vi "Measurement Logic.vi"() -> ()   [LabVIEW 2024, in "NIFgenSignalVoltageGeneration.lvlib"]
uses:
  NIFgenSignalVoltageGeneration.lvlib
  Measurement Configuration.ctl
  Measurement Results.ctl
  <vilib>/MeasurementLink/MeasurementLink Measurement Server/Measure Call Context/Measure Call Context.lvclass
  <instrlib>/niFgen/niFgen.llb/niFgen Output Mode.ctl
  <vilib>/MeasurementLink/MeasurementLink niFGEN/Initialize Sessions - 1Sess.vi
  <vilib>/MeasurementLink/MeasurementLink Session Management V1/Session Reservation/Session Reservation.lvclass
  <vilib>/MeasurementLink/MeasurementLink niFGEN/MeasurementLink niFGEN.lvlib
panel:
  out "Generated Waveform":waveform(dbl)(graph)
  out "actual duration":dbl
  out "measure call context out":refnum<class "Measure Call Context.lvclass">
  in  "measure call context in":refnum<class "Measure Call Context.lvclass">
  out "measurement results":T1
  in  "measurement configuration":T2={"Pin Name"="Pin1", "Generation Time (s)"=0.0, "Voltage Offset (V)"=0.0, "Sample Rate (Hz)"=1000000.0, "Frequency (Hz)"=200000.0, "Amplitude (V)"=1.0, "Waveform"=0} {"Waveform" items=["Sine"=0, "Square"=3]}
  out "error out":errorcluster
  in  "error in":errorcluster
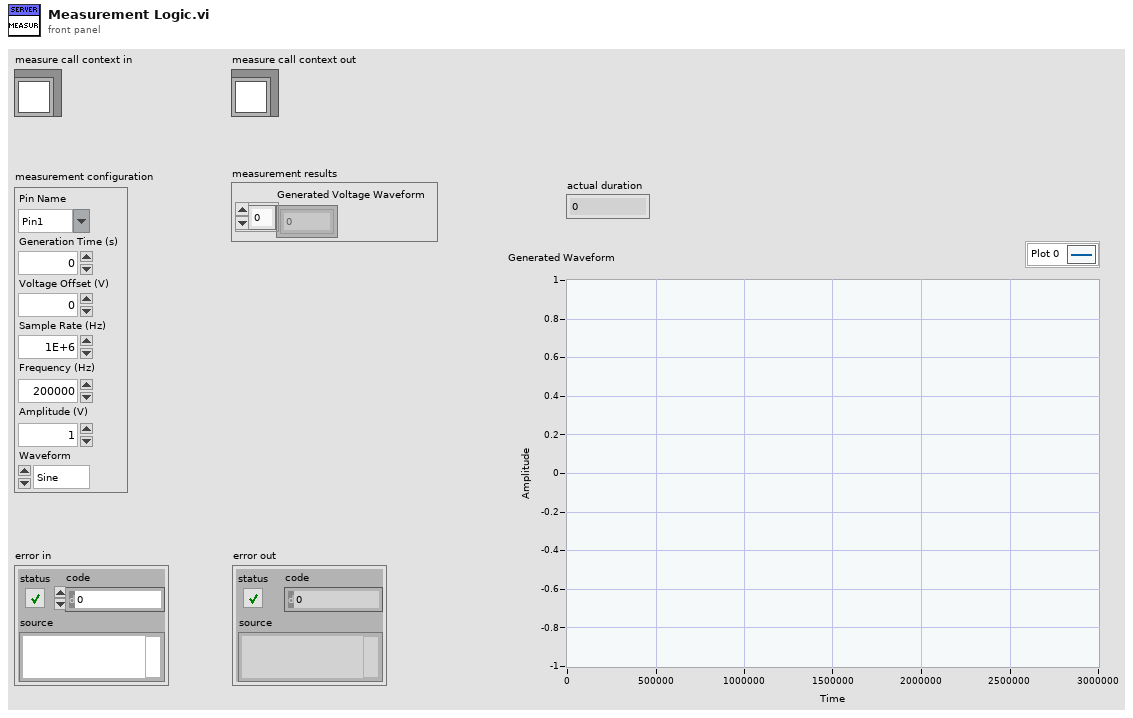
[diagram p1: front panel]
types:
  T1 = typedef "NIFgenSignalVoltageGeneration.lvlib/Measurement Results.ctl" = cluster{"Generated Voltage Waveform":dbl[]}
  T2 = typedef "NIFgenSignalVoltageGeneration.lvlib/Measurement Configuration.ctl" = cluster{"Pin Name":string, "Generation Time (s)":dbl, "Voltage Offset (V)":dbl, "Sample Rate (Hz)":dbl, "Frequency (Hz)":dbl, "Amplitude (V)":dbl, "Waveform":i32}
  T3 = typedef "niFgen Output Mode.ctl" = u32
  T4 = cluster{"Waveform":i32, "Amplitude (V)":dbl, dbl}
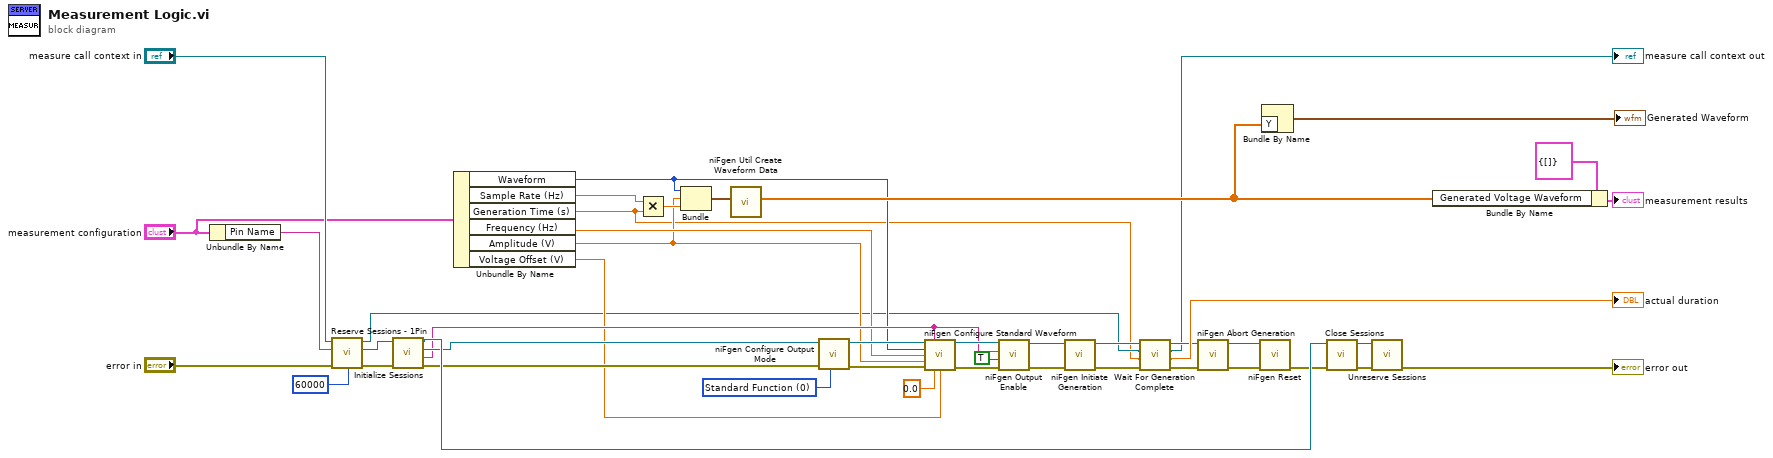
[diagram p0: block diagram]
diagram:
  w40 = T3 0 items=["Standard Function", "Frequency List", "Arbitrary Waveform", "Arbitrary Sequence", "Script"] ("Output Mode (default: 0=Standard Function)")
  n1 = Unbundle By Name("measurement configuration") -> ("Pin Name"=w18:string)
  n2 = call <vilib>:"Reserve Sessions - 1Pin.vi"("timeout (ms)"=60000, "error in"="error in", "pin or relay name"=w18, "measurement context in"="measure call context in") -> ("error out"=w43:errorcluster, "session reservation out"=w42:refnum<class "Session Reservation.lvclass">, "measurement context out"=w7:refnum<class "Measure Call Context.lvclass">)  [unwired: 5 in]
  n3 = call-poly <vilib>:"Initialize Sessions.vi"("error in"=w43, "session reservation in"=w42) -> ("error out"=w36:errorcluster, "channel list"=w23:string, "session"=w35:refnum<k15>, "session reservation out"=w37:refnum<class "Session Reservation.lvclass">)  [unwired: 6 in]
  n4 = Unbundle By Name("measurement configuration") -> ("Waveform"=w9:i32, "Sample Rate (Hz)"=w21:dbl, "Generation Time (s)"=w3:dbl, "Frequency (Hz)"=w16:dbl, "Amplitude (V)"=w15:dbl, "Voltage Offset (V)"=w14:dbl)
  n5 = Multiply(x=w21, y=w3) -> (x*y=w22:dbl)
  n6 = Bundle("Waveform"=w9, "Amplitude (V)"=w15, w22) -> (w20:T4)  [unwired: 1 in]
  n7 = call <instrlib>:"niFgen Util Create Waveform Data.vi"("Waveform"=w20) -> ("Waveform Data"=w13:dbl[])  [unwired: 10 in]
  n8 = call <instrlib>:"niFgen Configure Output Mode.vi"("error in (no error)"=w36, "Output Mode (default: 0=Standard Function)"=w40, "Instrument Handle"=w35) -> ("error out"=w26:errorcluster, "Instrument Handle Out"=w27:refnum<k15>)  [unwired: 6 in]
  n9 = call <instrlib>:"niFgen Configure Standard Waveform.vi"("Instrument Handle"=w27, "Channel Name"=w23, "Waveform"=w9, "Frequency"=w16, "Amplitude"=w15, "error in (no error)"=w26, "Start Phase"=0.0, "DC Offset"=w14) -> ("Instrument Handle Out"=w25:refnum<k15>, "error out"=w24:errorcluster)  [unwired: 6 in]
  n10 = call <instrlib>:"niFgen Output Enable.vi"("error in (no error)"=w24, "Output Enable (default: True)"=TRUE, "Channel Name"=w23, "Instrument Handle"=w25) -> ("error out"=w31:errorcluster, "Instrument Handle Out"=w30:refnum<k15>)  [unwired: 6 in]
  n11 = call <instrlib>:"niFgen Initiate Generation.vi"("error in (no error)"=w31, "Instrument Handle"=w30) -> ("error out"=w6:errorcluster, "Instrument Handle Out"=w8:refnum<k15>)  [unwired: 8 in]
  n12 = call "Wait For Generation Complete.vi"("error in"=w6, "duration"=w3, "measurement context in"=w7, "instrument handle in"=w8) -> ("error out"=w5:errorcluster, "actual duration"=→"actual duration":dbl, "measurement context out"=→"measure call context out":refnum<class "Measure Call Context.lvclass">, "instrument handle out"=w2:refnum<k15>)  [unwired: 4 in]
  n13 = call <instrlib>:"niFgen Abort Generation.vi"("error in (no error)"=w5, "Instrument Handle"=w2) -> ("error out"=w33:errorcluster, "Instrument Handle Out"=w34:refnum<k15>)  [unwired: 8 in]
  n14 = call <instrlib>:"niFgen Reset.vi"("error in (no error)"=w33, "Instrument Handle"=w34) -> ("error out"=w32:errorcluster)  [unwired: 8 in, 1 out]
  n15 = Bundle By Name("Y"=w13) -> (→"Generated Waveform":waveform(dbl))  [unwired: 1 in]
  n16 = call <vilib>:"Close Sessions.vi"("error in"=w32, "session reservation in"=w37) -> ("error out"=w38:errorcluster, "session reservation out"=w39:refnum<class "Session Reservation.lvclass">)  [unwired: 8 in]
  n17 = call <vilib>:"Unreserve Sessions.vi"("error in"=w38, "session reservation in"=w39) -> ("error out"=→"error out":errorcluster)  [unwired: 9 in]
  n18 = Bundle By Name(cluster=T1 {"Generated Voltage Waveform"=[]} ("Measurement Results"), "Generated Voltage Waveform"=w13) -> (→"measurement results":T1)
